vi "Licor-alpha.vi"(8 "P [kPa]":dbl format="%#_13g", 9 "T [K]":dbl, 10 "Psi_i":dbl, 11 "Chi_i":dbl) -> (3 "absorptance_i":dbl)   [LabVIEW 2010]
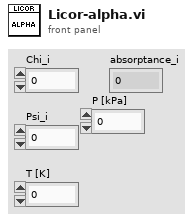
[diagram p1: front panel]
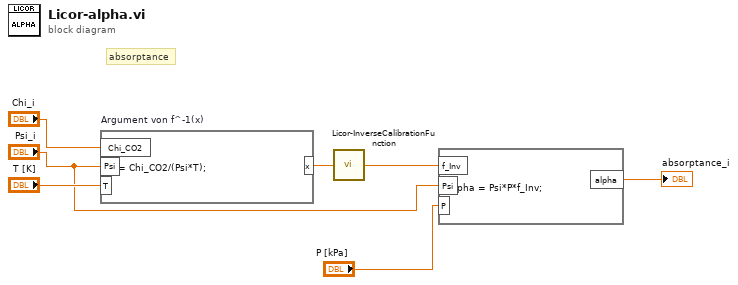
[diagram p0: block diagram]
diagram:
  # "absorptance"
  n1 = formula code="x = Chi_CO2/(Psi*T);" "Argument von f^-1(x)"("Chi_CO2"="Chi_i", "Psi"="Psi_i", "T"="T [K]") -> ("x"=w7:dbl)
  n2 = call "Licor-InverseCalibrationFunction.vi"("x"=w7) -> ("f_Inv(x)"=w4:dbl)  [unwired: 14 in]
  n3 = formula code="alpha = Psi*P*f_Inv;"("f_Inv"=w4, "Psi"="Psi_i", "P"="P [kPa]") -> ("alpha"=→"absorptance_i":dbl)
